vi "Pic Get Frame.vi"(8 "error in (no error)":errorcluster, 9 "frames":T2, 10 "Img Data indexed":cluster{"image data":T1, "bitmap":u32[][]}, 11 "LF2R IDE in":refnum<class "Main Panel.lvclass">) -> (0 "error out":errorcluster, 2 "Picture out":picture, 3 "LF2R IDE out":refnum<class "Main Panel.lvclass">)   [LabVIEW 2018, in "Main Panel.lvlib" / "Main Panel.lvclass"]
uses:
  Main Panel.lvclass
  Image Json Parser/Img Json Frames.ctl
  <vilib>/picture/picture.llb/imagedata.ctl
  <vilib>/picture/picture.llb/Draw True-Color Pixmap.vi
  Picture Process/Picture Process.lvclass
  Image Json Parser/Image Json Parser.lvclass
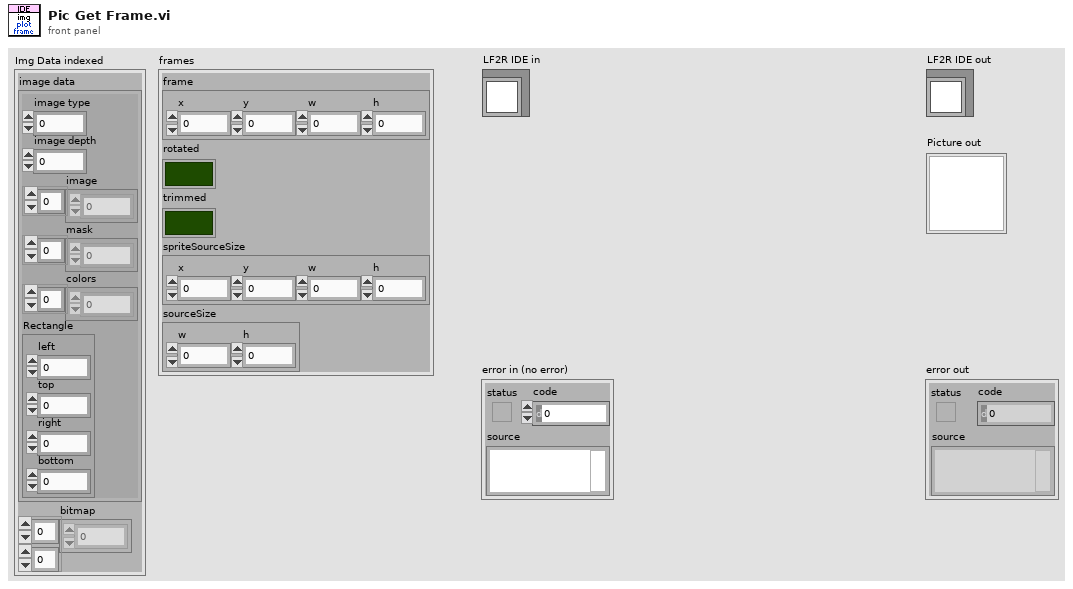
[diagram p1: front panel]
types:
  T1 = typedef "imagedata.ctl" = cluster{"image type":i32, "image depth":i32, "image":u8[], "mask":u8[], "colors":u32[], "Rectangle":cluster{"left":i16, "top":i16, "right":i16, "bottom":i16}}
  T2 = typedef "Image Json Parser.lvclass/Img Json Frames.ctl" = cluster{"frame":cluster{"x":i32, "y":i32, "w":i32, "h":i32}, "rotated":bool, "trimmed":bool, "spriteSourceSize":cluster{"x":i32, "y":i32, "w":i32, "h":i32}, "sourceSize":cluster{"w":i32, "h":i32}}
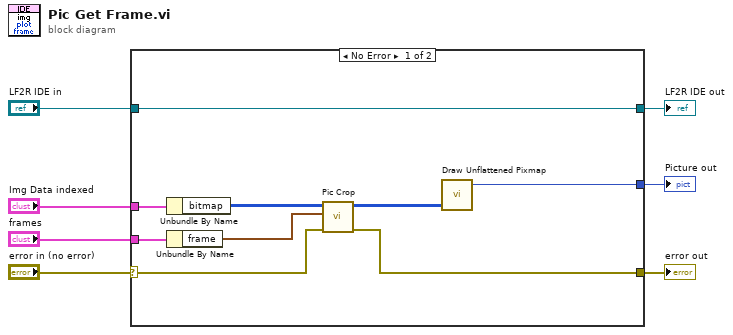
[diagram p0: block diagram]
diagram:
  n1 = case shown="No Error" "error in (no error)" {
    selector: "error in (no error)" -> [w12 w18]
    tunnel: [w11 w18] -> w6
    tunnel: [w10 w17] -> w4
    tunnel: "LF2R IDE in" -> [w10 w17]
    tunnel: "Img Data indexed" -> [w16 _]
    tunnel: "frames" -> [w15 _]
    tunnel: [w8 _] -> w1
    frame No Error {
      n2 = Unbundle By Name(w16) -> ("bitmap"=w14:u32[][])
      n3 = Unbundle By Name(w15) -> ("frame"=w13:cluster{"x":i32, "y":i32, "w":i32, "h":i32})
      n4 = call "Pic Crop.vi"("error in (no error)"=w12, "Position"=w13, "24-bit pixmap in"=w14) -> ("error out"=w11:errorcluster, "24-bit pixmap out"=w9:u32[][])  [unwired: 7 in]
      n5 = call-poly <vilib>:"Draw Unflattened Pixmap.vi"("data (RGB format)"=w9) -> ("new picture"=w8:picture)  [unwired: 8 in]
    }
    frame Error {
    }
  }
  "error out" <- w6
  "LF2R IDE out" <- w4
  "Picture out" <- w1
